vi "XY Coordinates.vi"(6 "axis info":T1, 7 "data history length (samples)":i32=100, 10 "Y coords":i32[](array[numeric]), 11 "X coords":i32[](array[numeric])) -> (1 "Y coords[]":i32[](array[numeric]), 2 "X coords[]":i32[](array[numeric]), 3 "XY Graph":cluster{i32[], i32[]}(graph)={[30426, 30426, 30426, 30426, 30426, 30426, 31206, 31206, 31206, 31206, 31206, 31206, 31206, 31206, 31206, 31206, 31206, 31206, 31206, 31986, 31986, 31986, 31986, 31986, 31206, 31206, 31206, 31206, 31206, 31206, 31206, 31206, 31206, 31206, 31206, 31206, 31206, 31206, 31206, 31206, 31206, 31206, 30426, 30426, 30426, 30426, 30426, 30426, 30426, 30426, 30426, 30426, 30426, 30426, 30426, 30426, 31206, 31206, 31206, 31206, 31206, 31206, 31206, 31206, 31206, 31206, 31206, 31206, 31206, 31206, 31206, 31206, 31206, 31206, 31206, 31206, 31206, 31206, 31206, 31206, 31206, 31206, 31206, 30426, 30426, 30426, 30426, 30426, 30426, 30426, 31206, 31206, 31206, 32246, 31466, 31466, 31466, 31466, 31466, 31466], [25745, 25745, 25745, 25745, 25745, 25745, 25745, 26525, 26525, 27306, 29386, 29386, 29386, 28086, 26785, 26785, 26785, 26785, 26785, 26785, 29646, 29646, 27045, 28086, 28086, 28086, 28086, 27306, 28346, 28346, 26785, 27826, 27826, 27566, 28346, 28346, 28346, 28346, 28346, 28346, 28346, 28346, 28346, 28346, 28346, 28346, 28346, 28346, 28346, 28346, 28346, 28346, 28346, 28346, 28346, 28346, 28346, 28346, 28346, 28346, 28346, 28346, 28346, 28346, 28346, 27566, 27566, 27566, 27566, 27566, 27566, 27566, 27566, 27566, 27566, 27566, 27566, 27566, 27566, 27566, 27566, 27566, 27566, 27566, 26785, 27566, 27566, 27566, 27566, 27566, 26265, 26265, 26265, 26265, 27045, 29126, 30426, 27826, 28606, 28606]})   [LabVIEW 2014, in "Joystick Fight Simulator.lvlib"]
doc: "Add new sample into size limited array, created to be used with feedbacks nodes outside to plot some last samples on XY graph."
uses:
  Joystick Fight Simulator.lvlib
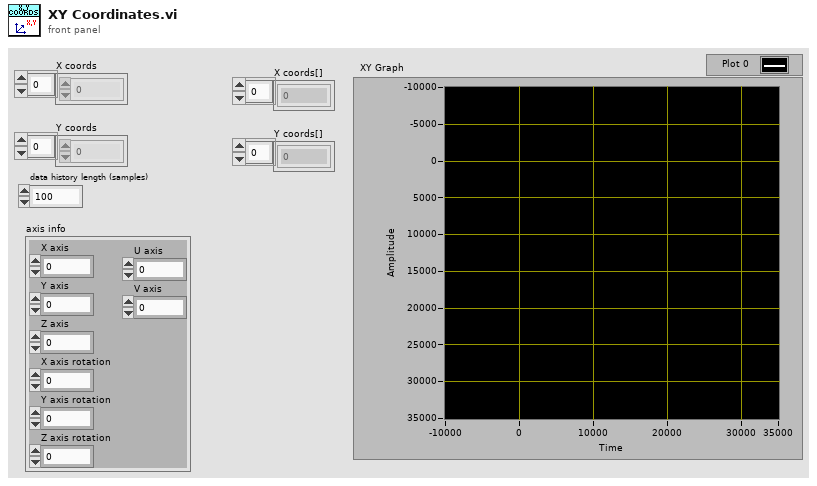
[diagram p1: front panel]
types:
  T1 = cluster{"X axis":i32, "Y axis":i32, "Z axis":i32, "X axis rotation":i32, "Y axis rotation":i32, "Z axis rotation":i32, "U axis":i32, "V axis":i32}
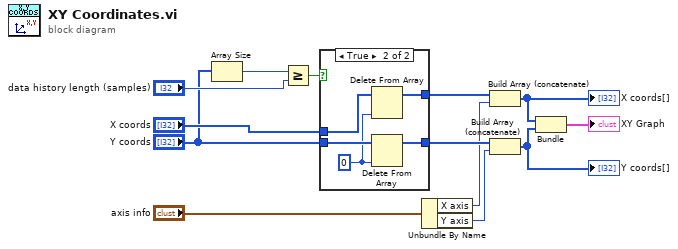
[diagram p0: block diagram]
diagram:
  n1 = Array Size(array="Y coords") -> (size(s)=w13:i32)
  n2 = Greater Or Equal?(x=w13, y="data history length (samples)") -> (x >= y?=w7:bool)
  n3 = case shown="True" w7 {
    tunnel: "Y coords" -> [w14 w19]
    tunnel: "X coords" -> [w15 w20]
    tunnel: [w14 w17] -> w10
    tunnel: [w15 w18] -> w11
    frame False {
    }
    frame True {
      w16 = 0 ("index")
      n4 = Delete From Array(array=w20, index=w16) -> (array with subset deleted=w18:i32[])  [unwired: 1 in, 1 out]
      n5 = Delete From Array(array=w19, index=w16) -> (array with subset deleted=w17:i32[])  [unwired: 1 in, 1 out]
    }
  }
  n6 = Unbundle By Name("axis info") -> ("X axis"=w3:i32, "Y axis"=w4:i32)
  n7 = Build Array (concatenate)(w11, w3) -> (w1:i32[])
  "X coords[]" <- w1
  n8 = Build Array (concatenate)(w10, w4) -> (w5:i32[])
  "Y coords[]" <- w5
  n9 = Bundle(w1, w5) -> (→"XY Graph":cluster{i32[], i32[]})  [unwired: 1 in]
